vi "MCL C Focus Get Focus Mode.vi"(8 "error in (no error)":errorcluster, 10 "handle":i32, 11 "focusLocked":i32) -> (0 "error out":errorcluster, 2 "function return":i32, 3 "focusLocked out":i32)   [LabVIEW 2014, in "Madlib.lvlib"]
doc: "MADLIB_API int MCL_CFocusGetFocusMode(int *focusLocked, int handle);"
uses:
  <userlib>/Lambda2/lib/Madlib/Madlib.lvlib
  <userlib>/Lambda2/lib/Madlib/Madlib.dll
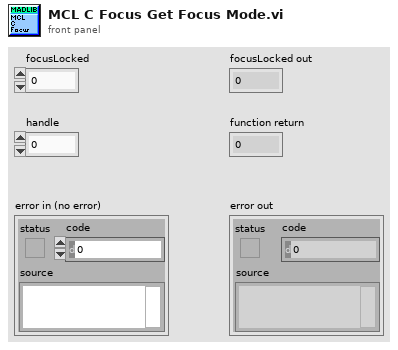
[diagram p1: front panel]
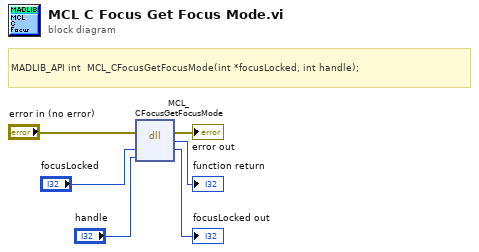
[diagram p0: block diagram]
diagram:
  # "MADLIB_API\tint\t\tMCL_CFocusGetFocusMode(int *focusLocked, int handle);"
  n1 = dll-call lib="C:/Program Files (x86)/National Instruments/LabVIEW 2014/user.lib/Lambda2/lib/Madlib/Madlib.*" fn="MCL_CFocusGetFocusMode"(error in="error in (no error)", "focusLocked"="focusLocked", "handle"="handle") -> (error out=→"error out":errorcluster, →"function return":i32, "focusLocked"=→"focusLocked out":i32)  [unwired: 3 in, 1 out]
